vi "Actor Template_Launch.vi"(9 "Timeout":i32=1000 format="%dmsec", 11 "error in":errorcluster) -> (4 "FTW Actor Connector":refnum<class "Actor Template.lvclass">, 6 "Initialized Response":string, 8 "Instance Inbox Address":string, 10 "Instance Publisher Address":string, 15 "error out":errorcluster)   [LabVIEW 2013, in "Actor Template.lvclass"]
uses:
  Actor Template.lvclass
  src/Connector/FTW-ActorConnector.lvclass
  Core/Actor Template-Core.lvclass
panel:
  in  "Boolean":bool
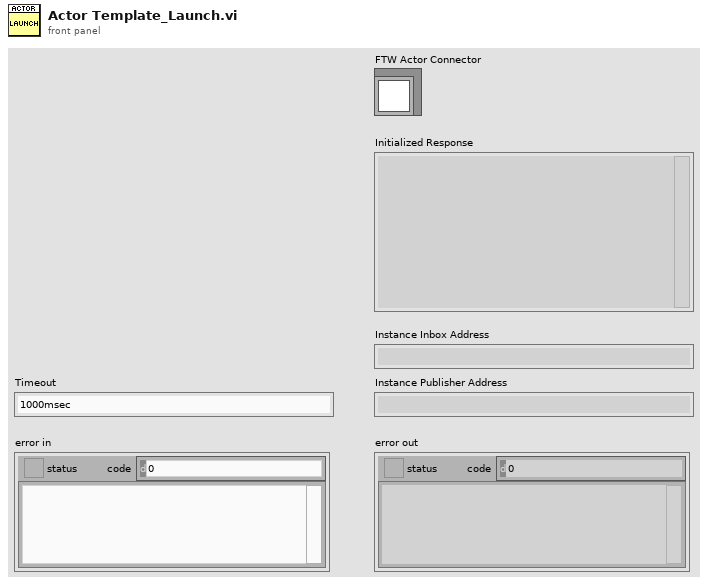
[diagram p1: front panel]
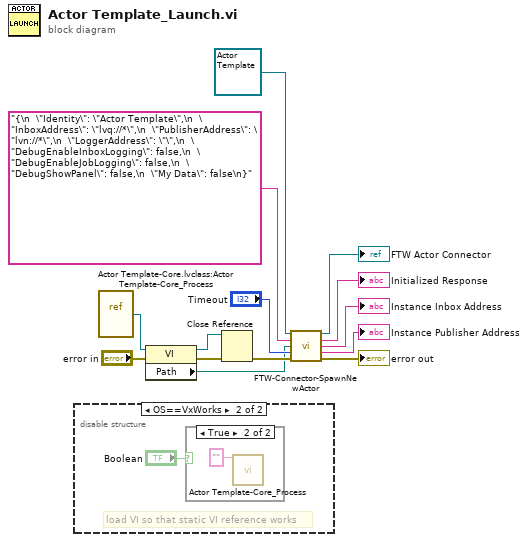
[diagram p0: block diagram]
diagram:
  n1 = disable-structure shown="OS==VxWorks" {
    frame condition #0 (active) {
    }
    frame condition #1 {
      # "load VI so that static VI reference works"
      n2 = case shown="True" "Boolean" {
        frame False {
        }
        frame True {
          n3 = call "Actor Template-Core_Process.vi"("FTW Actor Instance Configuration"="") -> ()  [unwired: 14 in, 1 out]
        }
      }
    }
  }
  n4 = vi-ref "Actor Template-Core.lvclass:Actor Template-Core_Process.vi"() -> (w6:refnum<vi>)
  n5 = property class="VI"(reference=w6, error in="error in") -> (reference out=w5:refnum<vi>, error out=w4:errorcluster, "Path"=w1:path)
  n6 = Close Reference(reference=w5, error in (no error)=w4) -> (error out=w2:errorcluster)
  n7 = call "FTW-Connector-SpawnNewActor.vi"("FTW Actor Connector Type"=refnum<class "Actor Template.lvclass"> refnum ("TTK_Splashscreen.lvclass"), "Configuration"="{\n  \"Identity\": \"Actor Template\",\n  \"InboxAddress\": \"lvq://*\",\n  \"PublisherAddress\": \"lvn://*\",\n  \"LoggerAddress\": \"\",\n  \"DebugEnableInboxLogging\": false,\n  \"DebugEnableJobLogging\": false,\n  \"DebugShowPanel\": false,\n  \"My Data\": false\n}", "Actor VI Filepath"=w1, "Timeout"="Timeout", "error in"=w2) -> ("FTW Actor Connector"=→"FTW Actor Connector":refnum<class "Actor Template.lvclass">, "Initialized Response"=→"Initialized Response":string, "Instance Inbox Address"=→"Instance Inbox Address":string, "Instance Publisher Address"=→"Instance Publisher Address":string, "error out"=→"error out":errorcluster)  [unwired: 6 in]
